vi "dotNetTick2LvTimestamp.vi"(3 ".NetTick":i64=635841651030010000) -> (1 "time stamp":timestamp)   [LabVIEW 2011, in "Konvolucio MCAN120803.lvlib"]
uses:
  <instrlib>/Konvolucio MCAN120803/Konvolucio MCAN120803.lvlib
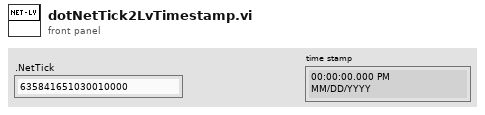
[diagram p1: front panel]
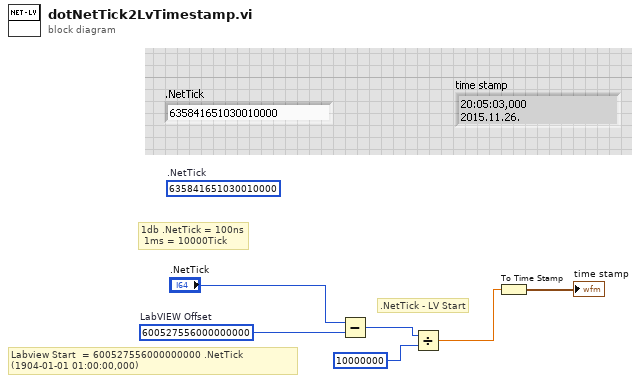
[diagram p0: block diagram]
diagram:
  w3 = i64 600527556000000000  # LabVIEW Offset
  (unwired) i64 635841651030010000  # .NetTick
  # ".NetTick - LV Start"
  # "1db .NetTick = 100ns\n 1ms = 10000Tick"
  # "Labview Start  = 600527556000000000 .NetTick\n(1904-01-01 01:00:00,000)"
  n1 = Subtract(x=".NetTick", y=w3) -> (x-y=w5:i64)
  n2 = Divide(x=w5, y=i64 10000000) -> (x/y=w1:dbl)
  n3 = To Time Stamp(1:w1) -> (0:→"time stamp":timestamp)
